vi "ADC_get_point.vi"(2 "Readout parameter":T1, 3 "Integration time (ms)":u32) -> (0 "data":dbl[](array[numeric]))   [LabVIEW 2013]
uses:
  <vilib>/DAQmx/read.llb/DAQmx Read (Analog 2D DBL NChan NSamp).vi
  <vilib>/Analysis/baseanly.llb/A x Vector.vi
  <vilib>/DAQmx/miscellaneous.llb/DAQmx Fill In Error Info.vi
  <vilib>/Analysis/NI_AALBase.lvlib
  <resource>/objmgr/daqmx.rc
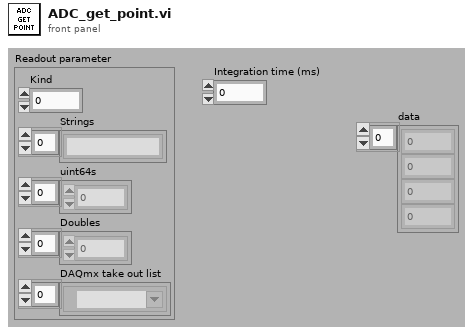
[diagram p1: front panel]
types:
  T1 = cluster{"Kind":u16, "Strings":string[], "uint64s":u64[], "Doubles":dbl[], "DAQmx take out list":refnum<k21>[]}
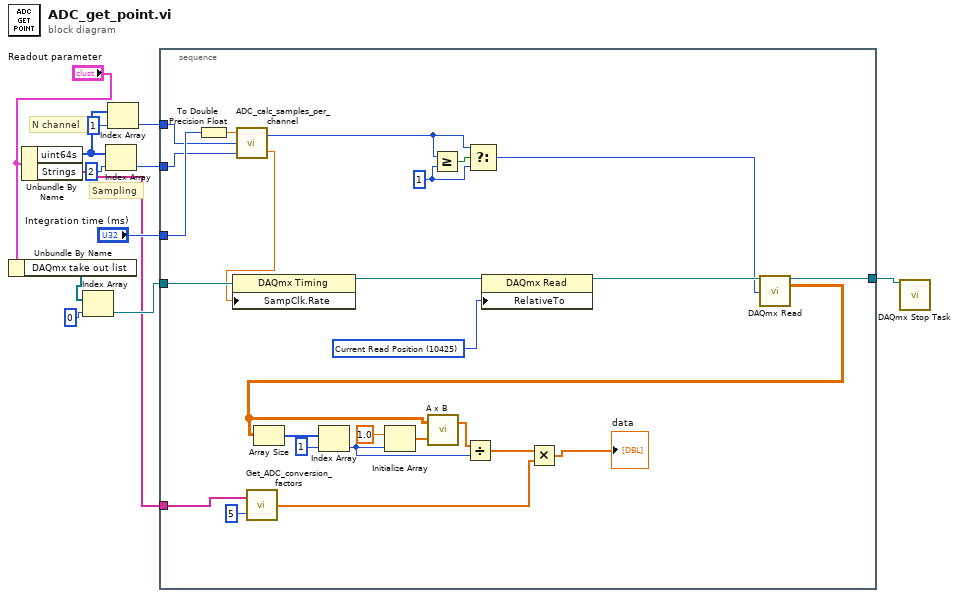
[diagram p0: block diagram]
diagram:
  # "Sampling"
  # "N channel"
  n1 = Unbundle By Name("Readout parameter") -> ("DAQmx take out list"=w4:refnum<k21>[])
  n2 = Unbundle By Name("Readout parameter") -> ("uint64s"=w12:u64[], "Strings"=w1:string[])
  n3 = Index Array(array=w4, index=0) -> (element=w2:refnum<k21>)
  n4 = Index Array(array=w12, index=2) -> (element=w9:u64)
  n5 = Index Array(array=w12, index=1) -> (element=w8:u64)
  n6 = stacked-sequence {
    tunnel: w9 -> [w16]
    tunnel: w8 -> [w17]
    tunnel: "Integration time (ms)" -> [w36]
    tunnel: w2 -> [w32]
    tunnel: [w23] -> w6
    tunnel: w1 -> [w22]
    frame #0 {
      w33 = 10425 items=["First Sample"=10424, "Current Read Position"=10425, "Reference Trigger"=10426, "First Pretrigger Sample"=10427, "Most Recent Sample"=10428] ("RelativeTo")
      w37 = 1 ("y")
      n7 = To Double Precision Float(number=w36) -> (double precision float=w18:dbl)
      n8 = call "ADC_calc_samples_per_channel.vi"("Samplingrate"=w16, "Nchannel"=w17, "time per point (ms)"=w18) -> ("effective samplingrate"=w14:dbl, "samples to read"=w15:u32)
      n9 = property class="DAQmx Timing"(reference=w32, "SampClk.Rate"=w14) -> (reference out=w35:refnum<k21>)  [unwired: 1 in, 1 out]
      n10 = call "Get_ADC_conversion_factors.vi"("index"=5, "Strings"=w22) -> ("elements"=w20:dbl[])
      n11 = Greater Or Equal?(x=w15, y=w37) -> (x >= y?=w38:bool)
      n12 = Select(t=w15, s=w38, f=w37) -> (s? t:f=w31:u32)
      n13 = property class="DAQmx Read"(reference=w35, "RelativeTo"=w33) -> (reference out=w34:refnum<k21>)  [unwired: 1 in, 1 out]
      n14 = call-poly <vilib>:"DAQmx Read.vi"("task/channels in"=w34, "number of samples per channel"=w31) -> ("task out"=w23:refnum<k21>, "data"=w24:dbl[][])  [unwired: 11 in, 1 out]
      n15 = Array Size(array=w24) -> (size(s)=w28:i32[])
      n16 = Index Array(array=w28, index=1) -> (element=w25:i32)
      n17 = Initialize Array(1.0 ("element"), w25) -> (w29:dbl[])
      n18 = call-poly <vilib>:"A x B.vi"("Vector"=w29, "A"=w24) -> ("A x Vector"=w26:dbl[])  [unwired: 1 out]
      n19 = Divide(x=w26, y=w25) -> (x/y=w21:dbl[])
      n20 = Multiply(x=w21, y=w20) -> (x*y=→"data":dbl[])
    }
  }
  n21 = call <vilib>:"DAQmx Stop Task.vi"("task/channels in"=w6) -> ()  [unwired: 13 in, 2 out]
